vi "control.vi"() -> (0 "Control CCD":T3={"Numero de lecturas"=1, "tiempo de lectura (ms)"=100, "Exposure"=0.053229, "Valor Gamma"=1.0, "Ganancia"=33, "Opción"=enum."Imágen", "VISA resource name"="", "Enable Strobe (Disabled)"=FALSE} {"Ganancia" min=0 max=100; "Valor Gamma" min=1.0 max=2.2; "Exposure" min=5e-05 max=0.053229}, 1 "Config. voltaje y corriente":T4={"Voltaje inicial"=-10.0, "incremento"=0.5, " voltaje final"=10.0, "Function(0:Voltage)"=0, "Unit(V)"=0, "Measurement Function (0:Voltage)"=0, "VISA resource name"="USB0::0x05E6::0x2450::04435662::INSTR"} {"Measurement Function (0:Voltage)" items=["Voltage", "Current", "Power"]; "Unit(V)" items=["V", "mV", "kV", "A", "mA"]; "Function(0:Voltage)" items=["Voltage", "Current"]}, 2 "Control de espejos":T6={"Movimiento de spot en y"=0.78, "Movimiento de spot en x"=0.5255, "tipo "=enum."barrido", "yFin"=0.82, "Paso"=0.01, "xFin"=0.5655} {"Movimiento de spot en x" scale=-10.0..10.0; "Movimiento de spot en y" min=-10.0 max=10.0 scale=-10.0..10.0}, 3 "config. Polarizador":T5={"pos inic"=0.0, "pos.final"=5.0, "incremento"=1.0, "velocidad"=0.0}, 4 "Config. fotodiodo y potenciometro":T2={"tiempo. lect."=300, "num. med"=20, "tiempo. lectura"=0, "average rate"=0, "Readout Config"="POW", "Tipo de Medición"=enum."Lockin", "usar multimetro"=FALSE}, 5 "Laser":T1, 6 "corriente":bool, 7 "dispositivos":string[](array[string])=["ninguno", "ninguno", "voltaje", "ninguno", "ninguno"])   [LabVIEW 2016]
panel:
  in  "Dispositivo 5":string(combo)="ninguno"
  in  "Dispositivo 4":string(combo)="ninguno"
  in  "Dispositivo 3":string(combo)="ninguno"
  in  "Dispositivo 2":string(combo)="ninguno"
  in  "Dispositivo 1":string(combo)="ninguno"
  in  "medir corriente":bool
  in  "VISA resource name CCD":refnum<visa-resource-name>
  in  "stop":bool
  in  "usar multimetro":bool
  in  "VISA resource name voltaje":refnum<visa-resource-name>="USB0::0x05E6::0x2450::04435662::INSTR"
  in  "Combo Box 2":string(combo)="imagen"
  in  "Numeric":dbl=10.0 min=0.0 max=0.0
  in  "Opciones":string(combo)="Voltaje final"
  in  "dispositivo":string(combo)="Dispositivo 3"
  # "dispositivos control"
  # "dispositivos adquisicion"
  # "Amplificador Lock in"
  # "potenciometro"
  # "Espectro"
  # "Imágen"
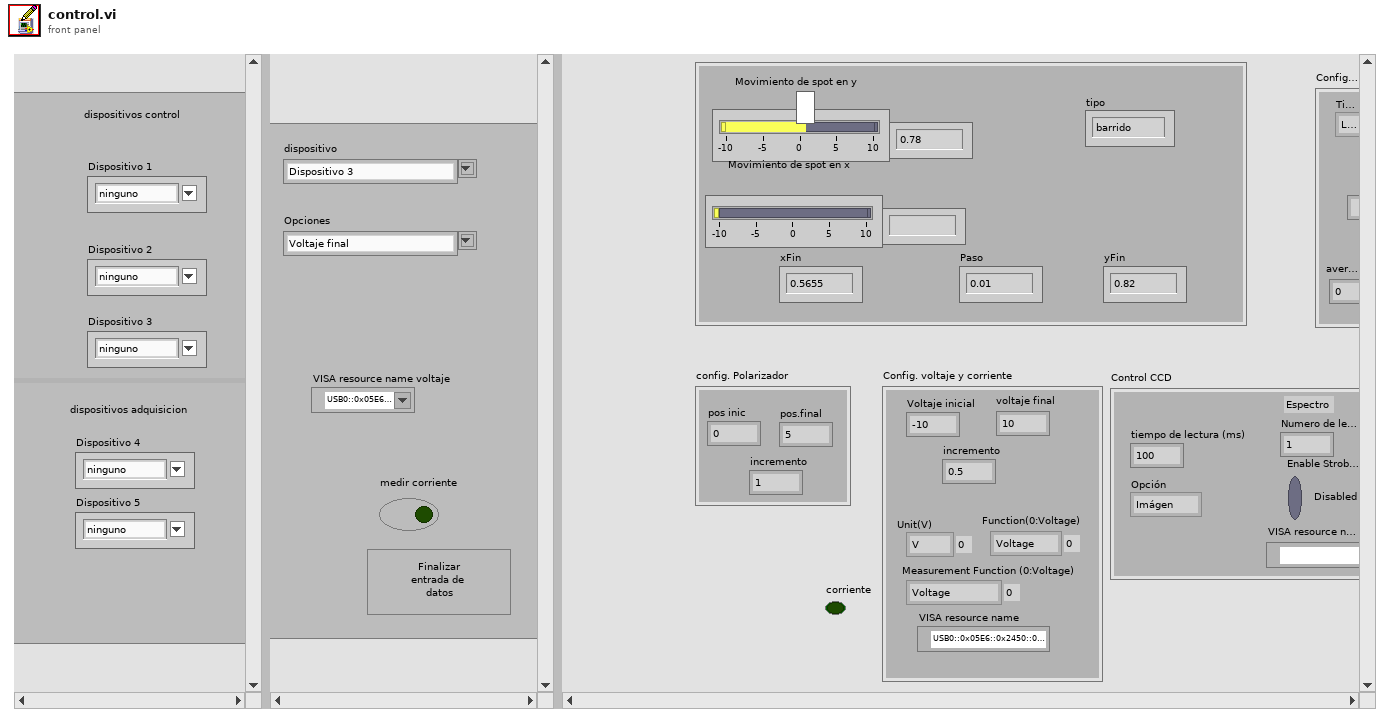
[diagram p1: front panel]
types:
  T1 = cluster{"corriente inicial":dbl, "temperatura":dbl, "corriente final ":dbl, "incremento":dbl}
  T2 = cluster{"tiempo. lect.":i32, "num. med":i32, "tiempo. lectura":i32, "average rate":i32, "Readout Config":string, "Tipo de Medición":enum16{"Lockin", "Lockin-potenciometro", "Potenciometro"}, "usar multimetro":bool}
  T3 = cluster{"Numero de lecturas":i32, "tiempo de lectura (ms)":u32, "Exposure":dbl, "Valor Gamma":dbl, "Ganancia":i64, "Opción":enum16{"Espectro", "Imágen"}, "VISA resource name":refnum<visa-resource-name>, "Enable Strobe (Disabled)":bool}
  T4 = cluster{"Voltaje inicial":dbl, "incremento":dbl, " voltaje final":dbl, "Function(0:Voltage)":u16, "Unit(V)":u16, "Measurement Function (0:Voltage)":u16, "VISA resource name":refnum<visa-resource-name>}
  T5 = cluster{"pos inic":dbl, "pos.final":dbl, "incremento":dbl, "velocidad":dbl}
  T6 = cluster{"Movimiento de spot en y":dbl, "Movimiento de spot en x":ext, "tipo ":enum16{"manual", "barrido"}, "yFin":dbl, "Paso":dbl, "xFin":dbl}
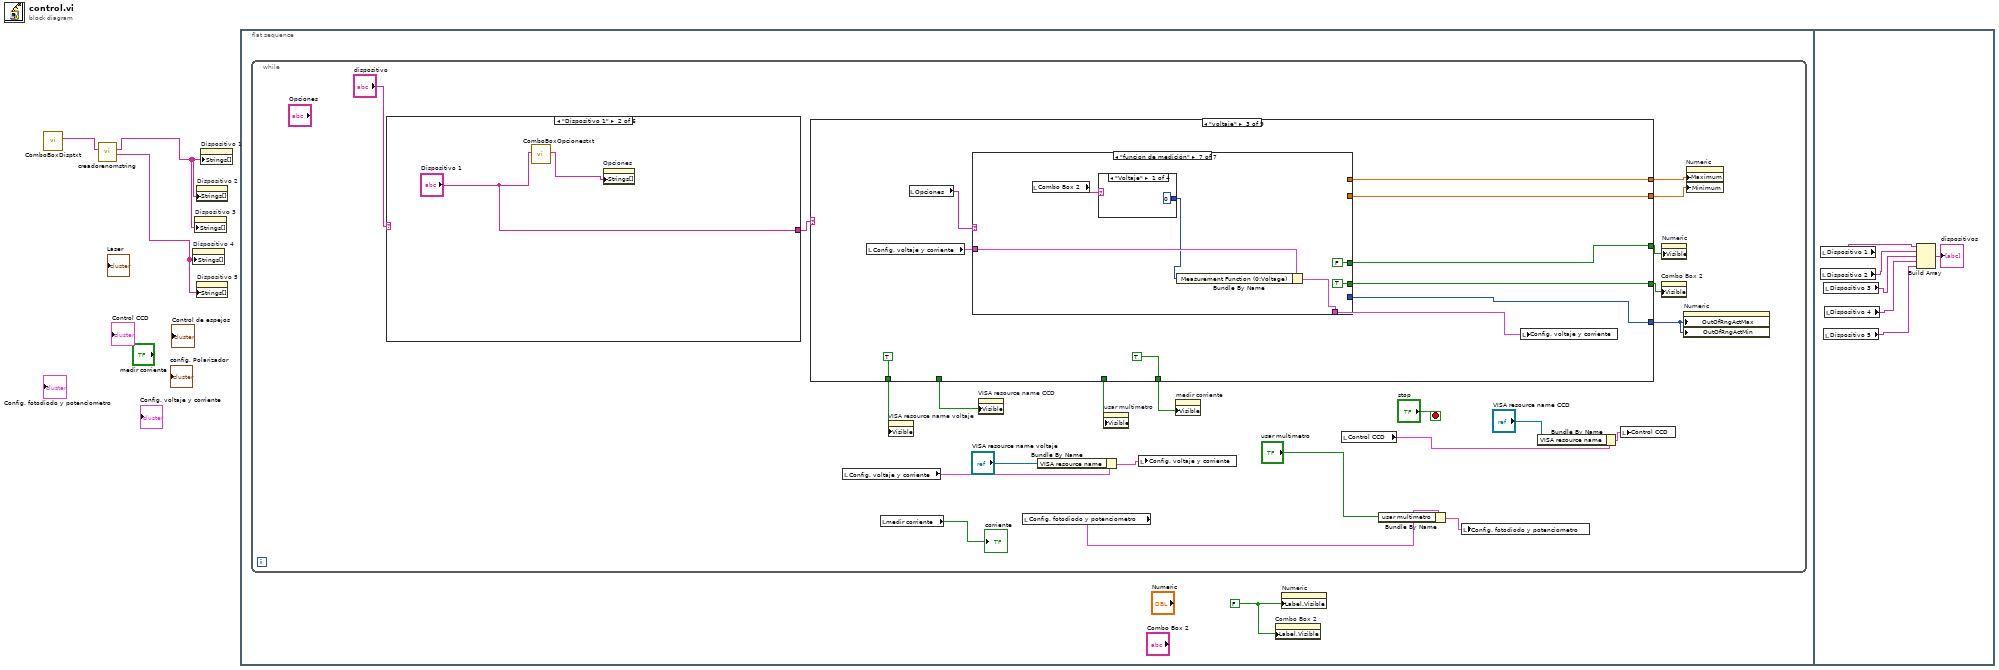
[diagram p0: block diagram]
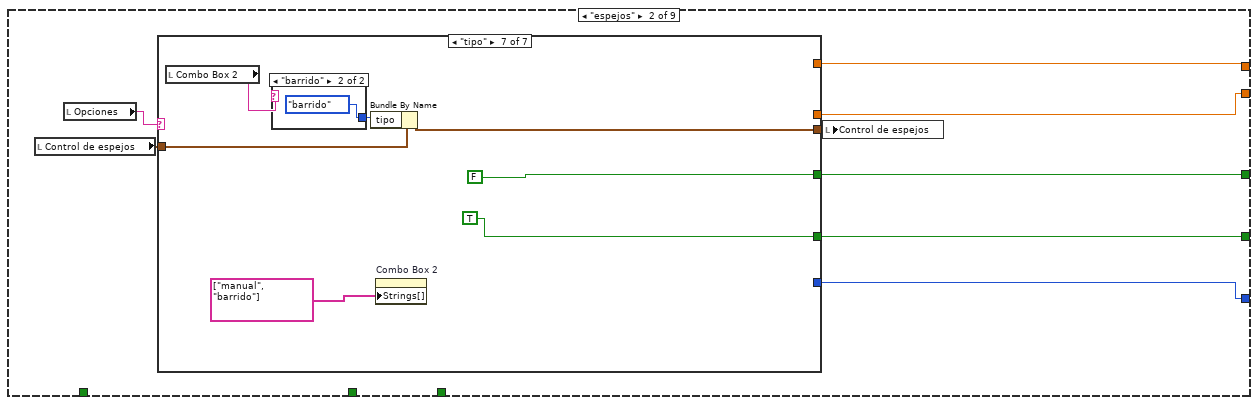
[diagram p3: hidden frame]
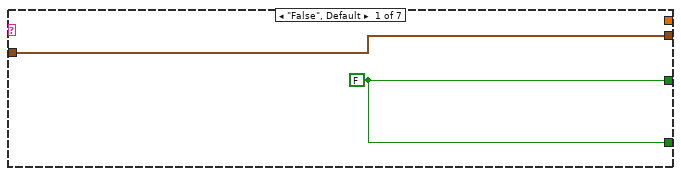
[diagram p4: hidden frame]
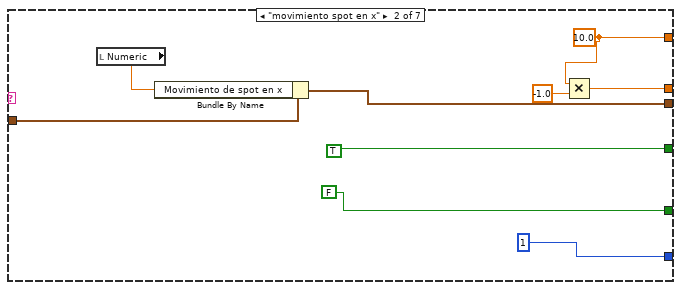
[diagram p5: hidden frame]
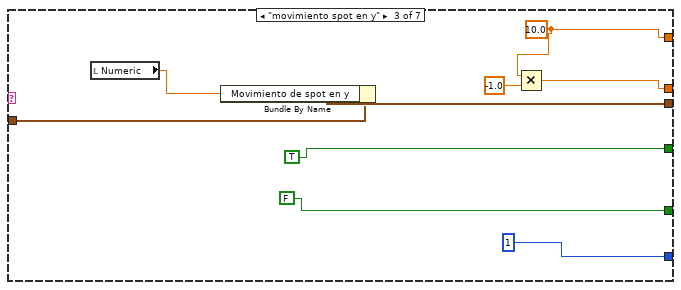
[diagram p6: hidden frame]
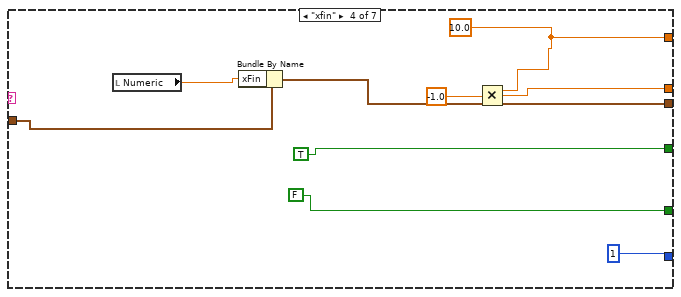
[diagram p7: hidden frame]
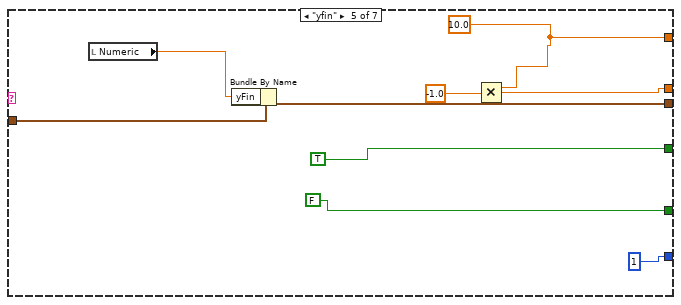
[diagram p8: hidden frame]
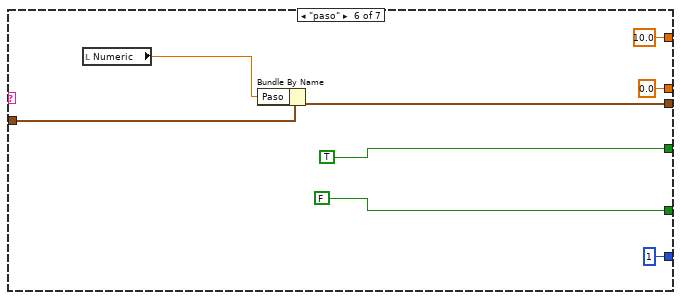
[diagram p9: hidden frame]
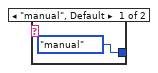
[diagram p10: hidden frame]
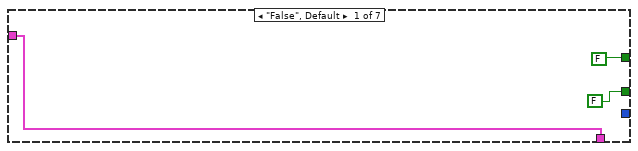
[diagram p11: hidden frame]
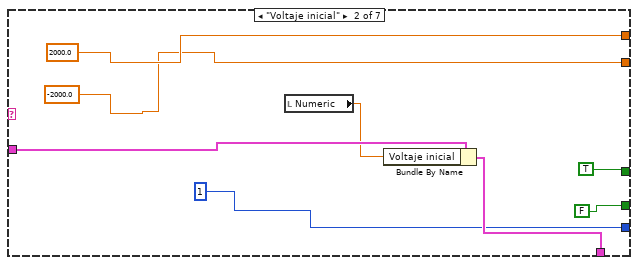
[diagram p12: hidden frame]
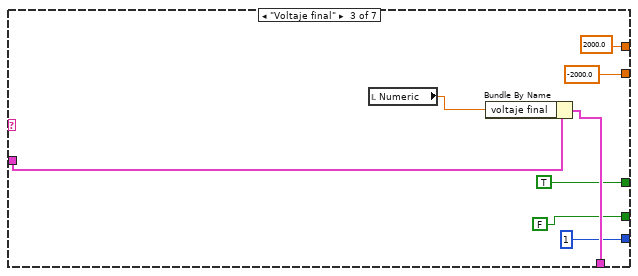
[diagram p13: hidden frame]
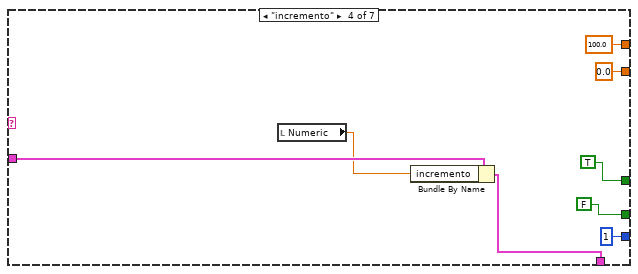
[diagram p14: hidden frame]
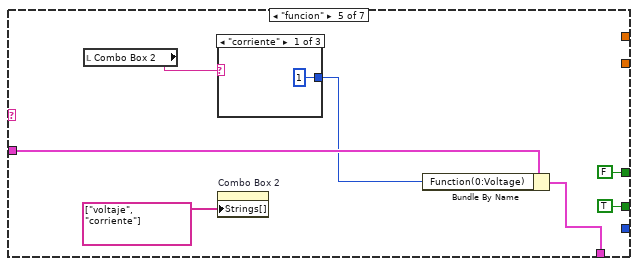
[diagram p15: hidden frame]
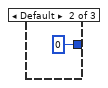
[diagram p16: hidden frame]
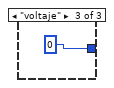
[diagram p17: hidden frame]
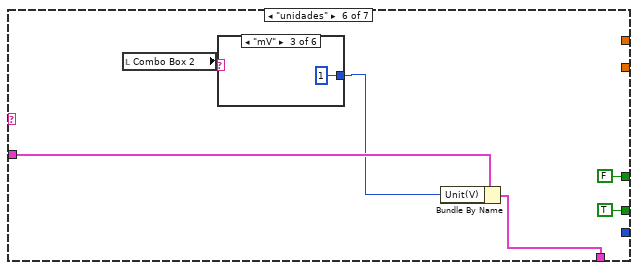
[diagram p18: hidden frame]
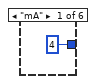
[diagram p19: hidden frame]
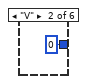
[diagram p20: hidden frame]
diagram:
  n1 = call "ComboBoxDisptxt.vi"() -> ("cadena"=w3:string[])  [unwired: 11 in]
  n2 = call "creadorenomstring.vi"("cadena"=w3) -> ("adquisicion"=w1:string[], "control"=w2:string[])  [unwired: 9 in]
  n3 = property on="Dispositivo 4" class="CmbBox"("Strings[]"=w1) -> ()  [unwired: 2 in, 2 out]
  n4 = property on="Dispositivo 3" class="CmbBox"("Strings[]"=w2) -> ()  [unwired: 2 in, 2 out]
  n5 = property on="Dispositivo 2" class="CmbBox"("Strings[]"=w2) -> ()  [unwired: 2 in, 2 out]
  n6 = property on="Dispositivo 5" class="CmbBox"("Strings[]"=w1) -> ()  [unwired: 2 in, 2 out]
  n7 = property on="Dispositivo 1" class="CmbBox"("Strings[]"=w2) -> ()  [unwired: 2 in, 2 out]
  n8 = flat-sequence {
    frame #0 {
      w4 = FALSE ("Label.Visible")
      n9 = while {
        stop <- "stop" stop-if-true
        n10 = case shown="\"Dispositivo 1\"" "dispositivo" {
          tunnel: [_ "Dispositivo 1" "Dispositivo 2" "Dispositivo 3" "Dispositivo 4" "Dispositivo 5"] -> w24
          frame "False", Default {
          }
          frame "Dispositivo 1" {
            n11 = call "ComboBoxOpcionestxt.vi"("dispositivo"="Dispositivo 1") -> ("array w/ subset deleted"=w376:string[])  [unwired: 10 in]
            n12 = property on="Opciones" class="CmbBox"("Strings[]"=w376) -> ()  [unwired: 2 in, 2 out]
          }
          frame "Dispositivo 2" {
            n13 = call "ComboBoxOpcionestxt.vi"("dispositivo"="Dispositivo 2") -> ("array w/ subset deleted"=w378:string[])  [unwired: 10 in]
            n14 = property on="Opciones" class="CmbBox"("Strings[]"=w378) -> ()  [unwired: 2 in, 2 out]
          }
          frame "Dispositivo 3" {
            n15 = call "ComboBoxOpcionestxt.vi"("dispositivo"="Dispositivo 3") -> ("array w/ subset deleted"=w380:string[])  [unwired: 10 in]
            n16 = property on="Opciones" class="CmbBox"("Strings[]"=w380) -> ()  [unwired: 2 in, 2 out]
          }
          frame "Dispositivo 4" {
            n17 = call "ComboBoxOpcionestxt.vi"("dispositivo"="Dispositivo 4") -> ("array w/ subset deleted"=w382:string[])  [unwired: 10 in]
            n18 = property on="Opciones" class="CmbBox"("Strings[]"=w382) -> ()  [unwired: 2 in, 2 out]
          }
          frame "Dispositivo 5" {
            n19 = call "ComboBoxOpcionestxt.vi"("dispositivo"="Dispositivo 5") -> ("array w/ subset deleted"=w384:string[])  [unwired: 10 in]
            n20 = property on="Opciones" class="CmbBox"("Strings[]"=w384) -> ()  [unwired: 2 in, 2 out]
          }
        }
        n21 = case shown="\"voltaje\"" w24 {
          tunnel: [_ w31 w96 w164 w236 w271 w306 w335 _] -> w23
          tunnel: [_ w30 w95 w163 w235 w270 w305 w336 _] -> w22
          tunnel: [_ _ _ TRUE _ _ _ _ _] -> w7
          tunnel: [_ _ TRUE _ _ _ _ _ _] -> w21
          tunnel: [_ _ _ _ _ TRUE ("Visible") TRUE ("Visible") _ _] -> w18
          tunnel: [_ w29 w93 w160 w234 w268 w303 w333 _] -> w16
          tunnel: [_ w28 w92 w161 w233 w267 w302 w332 _] -> w15
          tunnel: [_ w27 w91 w159 w232 w266 w301 w334 _] -> w14
          tunnel: [_ _ TRUE _ _ _ _ _ _] -> w6
          frame "False", Default {
          }
          frame "espejos" {
            n22 = local read "Control de espejos"() -> (w33:T6)
            n23 = local read "Opciones"() -> (w34:string)
            n24 = case shown="\"tipo\"" w34 {
              tunnel: w33 -> [w35 w42 w53 w60 w69 w77 w84]
              tunnel: [w35 w43 w54 w61 w70 w78 w85] -> w32
              tunnel: [w36 TRUE TRUE TRUE TRUE TRUE FALSE] -> w31
              tunnel: [w36 FALSE FALSE FALSE FALSE FALSE TRUE] -> w30
              tunnel: [_ w39 w48 w57 w66 10.0 ("Data Entry Limits:Maximum") _] -> w29
              tunnel: [_ w38 w47 w56 w65 0.0 _] -> w28
              tunnel: [_ u8 1 ("Response to Value Outside Limits:Maximum") u8 1 ("Response to Value Outside Limits:Maximum") u8 1 ("Response to Value Outside Limits:Maximum") u8 1 ("Response to Value Outside Limits:Maximum") u8 1 ("Response to Value Outside Limits:Maximum") _] -> w27
              frame "False", Default {
                w36 = FALSE
              }
              frame "movimiento spot en x" {
                w39 = 10.0 ("Data Entry Limits:Maximum")
                n25 = local read "Numeric"() -> (w41:dbl)
                n26 = Bundle By Name(cluster=w42, "Movimiento de spot en x"=w41) -> (w43:T6)
                n27 = Multiply(x=w39, y=-1.0) -> (x*y=w38:dbl)
              }
              frame "movimiento spot en y" {
                w48 = 10.0 ("Data Entry Limits:Maximum")
                n28 = local read "Numeric"() -> (w52:dbl)
                n29 = Bundle By Name(cluster=w53, "Movimiento de spot en y"=w52) -> (w54:T6)
                n30 = Multiply(x=w48, y=-1.0) -> (x*y=w47:dbl)
              }
              frame "xfin" {
                w57 = 10.0 ("Data Entry Limits:Maximum")
                n31 = local read "Numeric"() -> (w59:dbl)
                n32 = Bundle By Name(cluster=w60, "xFin"=w59) -> (w61:T6)
                n33 = Multiply(x=w57, y=-1.0) -> (x*y=w56:dbl)
              }
              frame "yfin" {
                w66 = 10.0 ("Data Entry Limits:Maximum")
                n34 = local read "Numeric"() -> (w68:dbl)
                n35 = Bundle By Name(cluster=w69, "yFin"=w68) -> (w70:T6)
                n36 = Multiply(x=w66, y=-1.0) -> (x*y=w65:dbl)
              }
              frame "paso" {
                n37 = local read "Numeric"() -> (w76:dbl)
                n38 = Bundle By Name(cluster=w77, "Paso"=w76) -> (w78:T6)
              }
              frame "tipo" {
                n39 = local read "Combo Box 2"() -> (w83:string)
                n40 = case shown="\"barrido\"" w83 {
                  tunnel: [enum16{"manual", "barrido"}."manual" ("tipo") enum16{"manual", "barrido"}."barrido" ("t")] -> w82
                  frame "manual", Default {
                  }
                  frame "barrido" {
                  }
                }
                n41 = Bundle By Name(cluster=w84, "tipo"=w82) -> (w85:T6)
                n42 = property on="Combo Box 2" class="CmbBox"("Strings[]"=string[] ["manual", "barrido"] ("Strings []")) -> ()  [unwired: 2 in, 2 out]
              }
            }
            n43 = local write "Control de espejos"(w32) -> ()
          }
          frame "voltaje" {
            n44 = local read "Config. voltaje y corriente"() -> (w98:T4)
            n45 = local read "Opciones"() -> (w99:string)
            n46 = case shown="\"funcion de medición\"" w99 {
              tunnel: w98 -> [w100 w108 w118 w123 w130 w139 w151]
              tunnel: [w100 w107 w117 w124 w128 w137 w150] -> w97
              tunnel: [FALSE TRUE TRUE TRUE FALSE FALSE FALSE] -> w96
              tunnel: [FALSE FALSE FALSE FALSE TRUE TRUE TRUE] -> w95
              tunnel: [_ 2000.0 ("Data Entry Limits:Maximum") 2000.0 ("Data Entry Limits:Maximum") 100.0 ("Data Entry Limits:Maximum") _ _ _] -> w93
              tunnel: [_ -2000.0 ("Data Entry Limits:Minimum") -2000.0 ("Data Entry Limits:Minimum") 0.0 ("Data Entry Limits:Minimum") _ _ _] -> w92
              tunnel: [_ u8 1 ("Response to Value Outside Limits:Maximum") u8 1 ("Response to Value Outside Limits:Maximum") u8 1 ("Response to Value Outside Limits:Maximum") _ _ _] -> w91
              frame "False", Default {
              }
              frame "Voltaje inicial" {
                n47 = local read "Numeric"() -> (w106:dbl)
                n48 = Bundle By Name(cluster=w108, "Voltaje inicial"=w106) -> (w107:T4)
              }
              frame "Voltaje final" {
                n49 = local read "Numeric"() -> (w114:dbl)
                n50 = Bundle By Name(cluster=w118, "voltaje final"=w114) -> (w117:T4)
              }
              frame "incremento" {
                n51 = local read "Numeric"() -> (w122:dbl)
                n52 = Bundle By Name(cluster=w123, "incremento"=w122) -> (w124:T4)
              }
              frame "funcion" {
                n53 = local read "Combo Box 2"() -> (w131:string)
                n54 = case shown="\"corriente\"" w131 {
                  tunnel: [1 0 0] -> w129
                  frame "corriente" {
                  }
                  frame Default {
                  }
                  frame "voltaje" {
                  }
                }
                n55 = property on="Combo Box 2" class="CmbBox"("Strings[]"=string[] ["voltaje", "corriente"] ("Strings []")) -> ()  [unwired: 2 in, 2 out]
                n56 = Bundle By Name(cluster=w130, "Function(0:Voltage)"=w129) -> (w128:T4)
              }
              frame "unidades" {
                n57 = local read "Combo Box 2"() -> (w140:string)
                n58 = case shown="\"mV\"" w140 {
                  tunnel: [4 0 1 3 0 2] -> w138
                  frame "mA" {
                  }
                  frame "V" {
                  }
                  frame "mV" {
                  }
                  frame "A" {
                  }
                  frame Default {
                  }
                  frame "kV " {
                  }
                }
                n59 = Bundle By Name(cluster=w139, "Unit(V)"=w138) -> (w137:T4)
              }
              frame "funcion de medición" {
                n60 = local read "Combo Box 2"() -> (w154:string)
                n61 = case shown="\"Voltaje\"" w154 {
                  tunnel: [0 0 1 2] -> w149
                  frame "Voltaje" {
                  }
                  frame Default {
                  }
                  frame "corriente" {
                  }
                  frame "potencia " {
                  }
                }
                n62 = Bundle By Name(cluster=w151, "Measurement Function (0:Voltage)"=w149) -> (w150:T4)
              }
            }
            n63 = local write "Config. voltaje y corriente"(w97) -> ()
          }
          frame "CCD" {
            n64 = local read "Opciones"() -> (w167:string)
            n65 = local read "Control CCD"() -> (w165:T3)
            n66 = case shown="\"Valor Gamma\"" w167 {
              tunnel: [w170 w179 w186 w191 w201 w213 w222 w230] -> w166
              tunnel: w165 -> [w170 w178 w187 w193 w203 w214 w223 w231]
              tunnel: [FALSE TRUE TRUE FALSE FALSE TRUE TRUE TRUE] -> w164
              tunnel: [FALSE FALSE FALSE TRUE TRUE FALSE FALSE FALSE] -> w163
              tunnel: [_ 0.0 5e-05 _ _ 1.0 0.0 1.0] -> w161
              tunnel: [_ 1000.0 0.0532 _ _ 2.2 100.0 100.0] -> w160
              tunnel: [_ u8 1 ("Response to Value Outside Limits:Maximum") u8 1 ("Response to Value Outside Limits:Maximum") _ _ u8 1 ("Response to Value Outside Limits:Maximum") u8 1 ("Response to Value Outside Limits:Maximum") u8 1 ("Response to Value Outside Limits:Maximum")] -> w159
              frame "False", Default {
              }
              frame "tiempo de lectura" {
                n67 = local read "Numeric"() -> (w174:dbl)
                n68 = To Long Integer(number=w174) -> (32bit integer=w175:i32)
                n69 = Bundle By Name(cluster=w178, "tiempo de lectura (ms)"=w175) -> (w179:T3)
              }
              frame "exposicion" {
                n70 = local read "Numeric"() -> (w185:dbl)
                n71 = Bundle By Name(cluster=w187, "Exposure"=w185) -> (w186:T3)
              }
              frame "Opción" {
                n72 = local read "Combo Box 2"() -> (w194:string)
                n73 = case shown="\"imagen\"" w194 {
                  tunnel: [0 1 0] -> w192
                  frame Default {
                  }
                  frame "imagen" {
                  }
                  frame "espectro" {
                  }
                }
                n74 = property on="Combo Box 2" class="CmbBox"("Strings[]"=string[] ["espectro", "imagen"] ("Strings []")) -> ()  [unwired: 2 in, 2 out]
                n75 = Bundle By Name(cluster=w193, "Opción"=w192) -> (w191:T3)
              }
              frame "Enable strobe" {
                n76 = local read "Combo Box 2"() -> (w204:string)
                n77 = case shown="\"deshabilitado\", Default" w204 {
                  tunnel: [FALSE TRUE] -> w202
                  frame "deshabilitado", Default {
                  }
                  frame "habilitado" {
                  }
                }
                n78 = property on="Combo Box 2" class="CmbBox"("Strings[]"=string[] ["habilitado", "deshabilitado"] ("Strings []")) -> ()  [unwired: 2 in, 2 out]
                n79 = Bundle By Name(cluster=w203, "Enable Strobe (Disabled)"=w202) -> (w201:T3)
              }
              frame "Valor Gamma" {
                n80 = local read "Numeric"() -> (w212:dbl)
                n81 = Bundle By Name(cluster=w214, "Valor Gamma"=w212) -> (w213:T3)
              }
              frame "Ganancia" {
                n82 = local read "Numeric"() -> (w220:dbl)
                n83 = To Long Integer(number=w220) -> (32bit integer=w221:i32)
                n84 = Bundle By Name(cluster=w223, "Ganancia"=w221) -> (w222:T3)
              }
              frame "Número de lecturas" {
                n85 = local read "Numeric"() -> (w229:dbl)
                n86 = Bundle By Name(cluster=w231, "Numero de lecturas"=w229) -> (w230:T3)
              }
            }
            n87 = local write "Control CCD"(w166) -> ()
          }
          frame "polarizador" {
            n88 = local read "config. Polarizador"() -> (w238:T5)
            n89 = local read "Opciones"() -> (w239:string)
            n90 = case shown="\"False\", Default" w239 {
              tunnel: w238 -> [w241 w247 w257 w265]
              tunnel: [w241 w246 w255 w261] -> w237
              tunnel: [w240 TRUE TRUE TRUE] -> w236
              tunnel: [w240 FALSE FALSE FALSE] -> w235
              tunnel: [_ 360.0 ("Data Entry Limits:Maximum") 360.0 ("Data Entry Limits:Maximum") 360.0 ("Data Entry Limits:Maximum")] -> w234
              tunnel: [_ 0.0 ("Data Entry Limits:Minimum") 0.0 ("Data Entry Limits:Minimum") -360.0 ("Data Entry Limits:Minimum")] -> w233
              tunnel: [_ u8 1 ("Response to Value Outside Limits:Minimum") u8 1 ("Response to Value Outside Limits:Maximum") u8 1 ("Response to Value Outside Limits:Maximum")] -> w232
              frame "False", Default {
                w240 = FALSE
              }
              frame "angulo inicial" {
                n91 = local read "Numeric"() -> (w245:dbl)
                n92 = Bundle By Name(cluster=w247, "pos inic"=w245) -> (w246:T5)
              }
              frame "angulo final" {
                n93 = local read "Numeric"() -> (w256:dbl)
                n94 = Bundle By Name(cluster=w257, "pos.final"=w256) -> (w255:T5)
              }
              frame "incremento" {
                n95 = local read "Numeric"() -> (w262:dbl)
                n96 = Bundle By Name(cluster=w265, "incremento"=w262) -> (w261:T5)
              }
            }
            n97 = local write "config. Polarizador"(w237) -> ()
          }
          frame "potenciometro" {
            n98 = local read "Config. fotodiodo y potenciometro"() -> (w273:T2)
            n99 = local read "Opciones"() -> (w274:string)
            n100 = case shown="\"average rate\"" w274 {
              tunnel: w273 -> [w277 w286 w291 w300]
              tunnel: [w277 w285 w290 w295] -> w272
              tunnel: [FALSE TRUE FALSE TRUE] -> w271
              tunnel: [FALSE FALSE TRUE FALSE] -> w270
              tunnel: [_ 10000.0 ("Data Entry Limits:Maximum") _ 10000.0 ("Data Entry Limits:Maximum")] -> w268
              tunnel: [_ 0.0 ("Data Entry Limits:Minimum") _ 0.0 ("Data Entry Limits:Minimum")] -> w267
              tunnel: [_ u8 1 ("Response to Value Outside Limits:Maximum") _ u8 1 ("Response to Value Outside Limits:Maximum")] -> w266
              frame "False", Default {
              }
              frame "average rate" {
                n101 = local read "Numeric"() -> (w283:dbl)
                n102 = To Long Integer(number=w283) -> (32bit integer=w284:i32)
                n103 = Bundle By Name(cluster=w286, "average rate"=w284) -> (w285:T2)
              }
              frame "readout config" {
                n104 = Bundle By Name(cluster=w291, "Readout Config"="POW") -> (w290:T2)
              }
              frame "tiempo de lectura" {
                n105 = local read "Numeric"() -> (w298:dbl)
                n106 = To Long Integer(number=w298) -> (32bit integer=w299:i32)
                n107 = Bundle By Name(cluster=w300, "tiempo. lectura"=w299) -> (w295:T2)
              }
            }
            n108 = local write "Config. fotodiodo y potenciometro"(w272) -> ()
          }
          frame "Lockin" {
            n109 = local read "Config. fotodiodo y potenciometro"() -> (w309:T2)
            n110 = local read "Opciones"() -> (w308:string)
            n111 = case shown="\"tiempo de lectura\"" w308 {
              tunnel: w309 -> [w311 w320 w329]
              tunnel: [w311 w319 w328] -> w307
              tunnel: [w310 TRUE TRUE] -> w306
              tunnel: [w310 FALSE FALSE] -> w305
              tunnel: [_ 10000.0 ("Data Entry Limits:Maximum") 10000.0 ("Data Entry Limits:Maximum")] -> w303
              tunnel: [_ 0.0 ("Data Entry Limits:Minimum") 0.0 ("Data Entry Limits:Minimum")] -> w302
              tunnel: [_ u8 1 ("Response to Value Outside Limits:Maximum") u8 1 ("Response to Value Outside Limits:Maximum")] -> w301
              frame "False", Default {
                w310 = FALSE
              }
              frame "tiempo de lectura" {
                n112 = local read "Numeric"() -> (w317:dbl)
                n113 = To Long Integer(number=w317) -> (32bit integer=w318:i32)
                n114 = Bundle By Name(cluster=w320, "tiempo. lect."=w318) -> (w319:T2)
              }
              frame "número de mediciones" {
                n115 = local read "Numeric"() -> (w326:dbl)
                n116 = To Long Integer(number=w326) -> (32bit integer=w327:i32)
                n117 = Bundle By Name(cluster=w329, "num. med"=w327) -> (w328:T2)
              }
            }
            n118 = local write "Config. fotodiodo y potenciometro"(w307) -> ()
          }
          frame "Laser" {
            n119 = local read "Opciones"() -> (w337:string)
            n120 = local read "Laser"() -> (w331:T1)
            n121 = case shown="\"corriente final\"" w337 {
              tunnel: [FALSE FALSE FALSE FALSE FALSE] -> w336
              tunnel: [FALSE TRUE TRUE TRUE TRUE] -> w335
              tunnel: [u8 1 ("Response to Value Outside Limits:Maximum") u8 1 ("Response to Value Outside Limits:Maximum") u8 1 ("Response to Value Outside Limits:Maximum") u8 1 ("Response to Value Outside Limits:Maximum") u8 1 ("Response to Value Outside Limits:Maximum")] -> w334
              tunnel: [70.0 0.01 0.1 0.1 0.1] -> w333
              tunnel: [-10.0 0.0 0.0 0.0 0.0] -> w332
              tunnel: w331 -> [w338 w346 w354 w367 w375]
              tunnel: [w338 w345 w353 w366 w374] -> w330
              frame "False", Default {
              }
              frame "temperatura" {
                n122 = local read "Numeric"() -> (w344:dbl)
                n123 = Bundle By Name(cluster=w346, "temperatura"=w344) -> (w345:T1)
              }
              frame "corriente inicial" {
                n124 = local read "Numeric"() -> (w352:dbl)
                n125 = Bundle By Name(cluster=w354, "corriente inicial"=w352) -> (w353:T1)
              }
              frame "corriente final" {
                n126 = local read "Numeric"() -> (w365:dbl)
                n127 = Bundle By Name(cluster=w367, "corriente final"=w365) -> (w366:T1)
              }
              frame "incremento" {
                n128 = local read "Numeric"() -> (w373:dbl)
                n129 = Bundle By Name(cluster=w375, "incremento"=w373) -> (w374:T1)
              }
            }
            n130 = local write "Laser"(w330) -> ()
          }
          frame "ninguno" {
          }
        }
        n131 = local read "Config. voltaje y corriente"() -> (w8:T4)
        n132 = local read "medir corriente"() -> (→"corriente":bool)
        n133 = property on="VISA resource name voltaje" class="VISAName"("Visible"=w21) -> ()  [unwired: 2 in, 2 out]
        n134 = property on="VISA resource name CCD" class="VISAName"("Visible"=w7) -> ()  [unwired: 2 in, 2 out]
        n135 = local read "Config. fotodiodo y potenciometro"() -> (w20:T2)
        n136 = Bundle By Name(cluster=w8, "VISA resource name"="VISA resource name voltaje") -> (w9:T4)
        n137 = property on="usar multimetro" class="Bool (strict)"("Visible"=w18) -> ()  [unwired: 2 in, 2 out]
        n138 = local write "Config. voltaje y corriente"(w9) -> ()
        n139 = property on="medir corriente" class="Bool (strict)"("Visible"=w6) -> ()  [unwired: 2 in, 2 out]
        n140 = local read "Control CCD"() -> (w12:T3)
        n141 = Bundle By Name(cluster=w20, "usar multimetro"="usar multimetro") -> (w19:T2)
        n142 = local write "Config. fotodiodo y potenciometro"(w19) -> ()
        n143 = Bundle By Name(cluster=w12, "VISA resource name"="VISA resource name CCD") -> (w11:T3)
        n144 = local write "Control CCD"(w11) -> ()
        n145 = property on="Combo Box 2" class="CmbBox"("Visible"=w22) -> ()  [unwired: 2 in, 2 out]
        n146 = property on="Numeric" class="DigNum (strict)"("Visible"=w23) -> ()  [unwired: 2 in, 2 out]
        n147 = property on="Numeric" class="DigNum (strict)"("OutOfRngActMax"=w14, "OutOfRngActMin"=w14) -> ()  [unwired: 2 in, 2 out]
        n148 = property on="Numeric" class="DigNum (strict)"("Maximum"=w16, "Minimum"=w15) -> ()  [unwired: 2 in, 2 out]
      }
      n149 = property on="Combo Box 2" class="CmbBox"("Label.Visible"=w4) -> ()  [unwired: 2 in, 2 out]
      n150 = property on="Numeric" class="DigNum (strict)"("Label.Visible"=w4) -> ()  [unwired: 2 in, 2 out]
    }
    frame #1 {
      n151 = local read "Dispositivo 1"() -> (w386:string)
      n152 = local read "Dispositivo 2"() -> (w387:string)
      n153 = local read "Dispositivo 3"() -> (w388:string)
      n154 = local read "Dispositivo 5"() -> (w390:string)
      n155 = local read "Dispositivo 4"() -> (w389:string)
      n156 = Build Array(w386, w387, w388, w389, w390) -> (→"dispositivos":string[])
    }
  }
